vi "GSP_Logger_Handler.vi"(4 "error in (no error)":errorcluster, 5 "Log":T1, 6 "Actions":T2(ring), 7 "Log File Path":path) -> (0 "error out":errorcluster)   [LabVIEW 2015]
doc: "Provides an interface to the Logger thread. See the actions below.\n\nLaunch - launch the logger, supplying the path to the log file\n\nOpen - Show the logger's front panel\n\nClose - Hide the logger's front panel\n\nLog - Record the event supplied by Log control\n\nShutdown - Shutdown the logger thread"
uses:
  LogItem.ctl
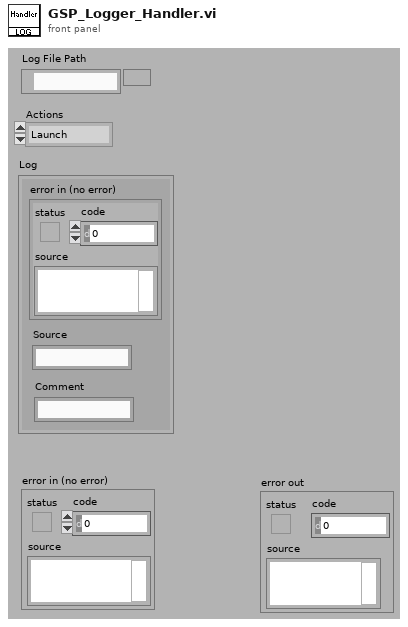
[diagram p1: front panel]
types:
  T1 = typedef "LogItem.ctl" = cluster{"error in (no error)":errorcluster, "Source":string, "Comment ":string}
  T2 = enum16{"Launch", "Log", "Open", "Close", "Shutdown"}
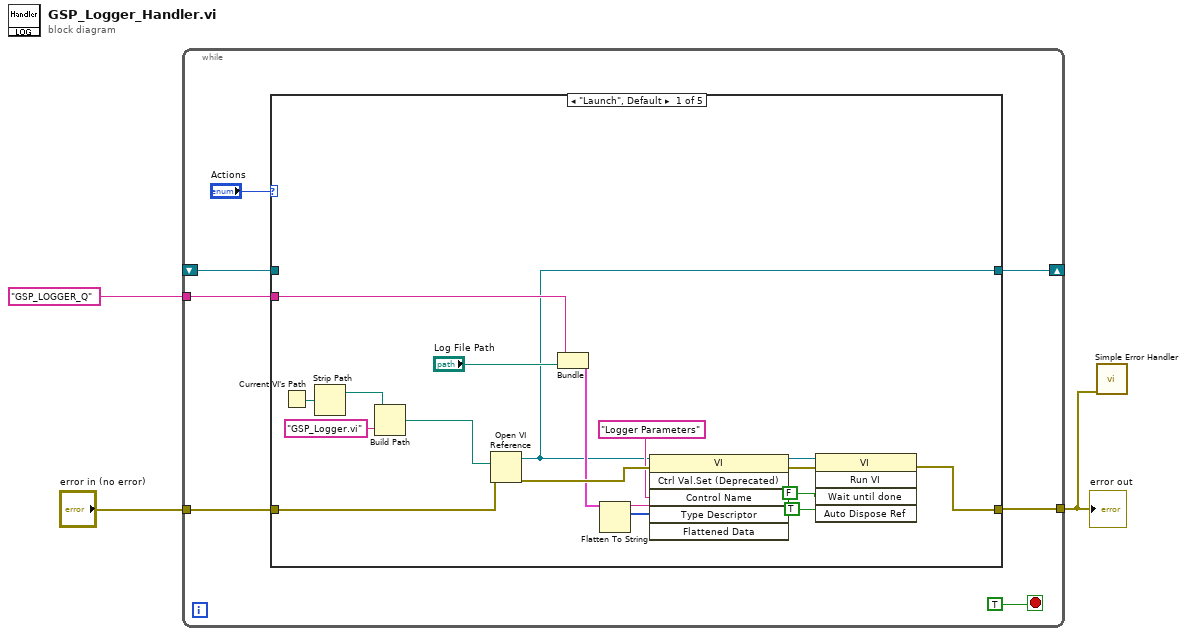
[diagram p0: block diagram]
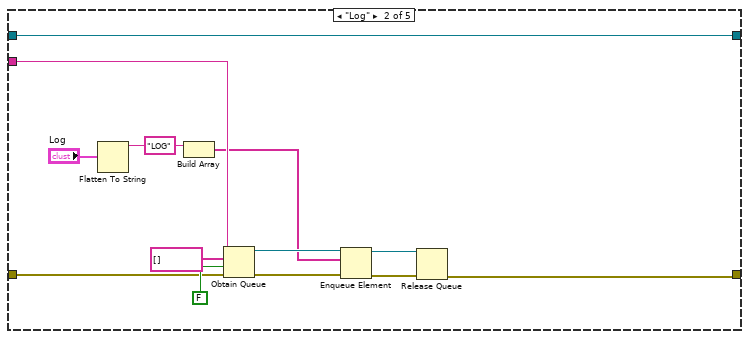
[diagram p2: hidden frame]
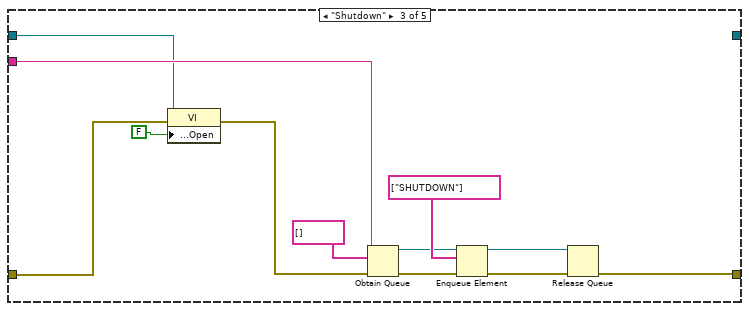
[diagram p3: hidden frame]
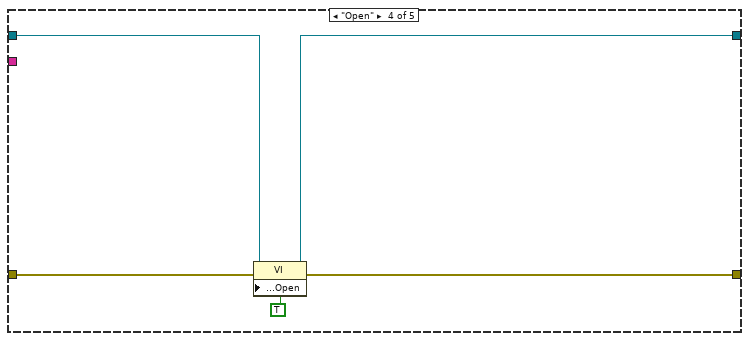
[diagram p4: hidden frame]
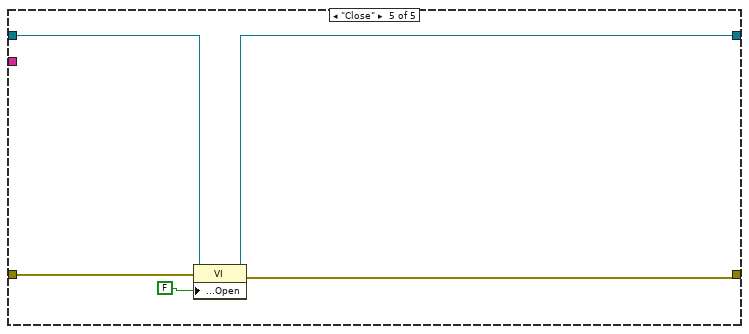
[diagram p5: hidden frame]
diagram:
  n1 = while {
    tunnel: "error in (no error)" -> [w7]
    tunnel: [w8] -> w1
    tunnel: "GSP_LOGGER_Q" -> [w6]
    shift-right: [w5] -> _
    shift-left: _ -> [w4]
    stop <- TRUE stop-if-true
    n2 = case shown="\"Launch\", Default" "Actions" {
      tunnel: w7 -> [w12 w40 w47 w58 w63]
      tunnel: [w14 w29 w43 w57 w60] -> w8
      tunnel: w6 -> [w13 w39 w52 _ _]
      tunnel: [w11 w32 _ w55 w61] -> w5
      tunnel: w4 -> [_ w32 w48 w56 w62]
      frame "Launch", Default {
        n3 = Current VI's Path() -> (path=w28:path)
        n4 = Strip Path(path=w28) -> (stripped path=w27:path)  [unwired: 1 out]
        n5 = Build Path(base path=w27, name or relative path="GSP_Logger.vi") -> (appended path=w25:path)
        n6 = Open VI Reference(vi path=w25, error in (no error)=w12) -> (vi reference=w11:refnum<vi>, error out=w24:errorcluster)  [unwired: 4 in]
        n7 = Bundle(w13, "Log File Path"="Log File Path") -> (w19:cluster{string, "Log File Path":path})  [unwired: 1 in]
        n8 = Flatten To String(anything=w19) -> (data string=w22:string, type string=w23:i16[])  [unwired: 3 in, 1 out]
        n9 = invoke class="VI" method="Ctrl Val.Set (Deprecated)"(reference=w11, error in=w24, "Control Name"="Logger Parameters", "Type Descriptor"=w23, "Flattened Data"=w22) -> (reference out=w18:refnum<vi>, error out=w17:errorcluster)  [unwired: 1 in, 4 out]
        n10 = invoke class="VI" method="Run VI"(reference=w18, error in=w17, "Wait until done"=FALSE, "Auto Dispose Ref"=TRUE) -> (error out=w14:errorcluster)  [unwired: 1 in, 4 out]
      }
      frame "Log" {
        n11 = Flatten To String(anything="Log") -> (data string=w35:string)  [unwired: 3 in, 2 out]
        n12 = Build Array("LOG" ("element"), w35) -> (w33:string[])
        n13 = Obtain Queue(name (unnamed)=w39, element data type=string[] [], create if not found? (T)=FALSE, error in (no error)=w40) -> (queue out=w38:refnum<queue>, error out=w37:errorcluster)  [unwired: 1 in, 1 out]
        n14 = Enqueue Element(queue=w38, element=w33, error in (no error)=w37) -> (queue out=w31:refnum<queue>, error out=w30:errorcluster)  [unwired: 1 in, 1 out]
        n15 = Release Queue(queue=w31, error in (no error)=w30) -> (error out=w29:errorcluster)  [unwired: 1 in, 2 out]
      }
      frame "Shutdown" {
        n16 = property class="VI"(reference=w48, error in=w47, "Front Panel Window:Open"=FALSE) -> (error out=w46:errorcluster)  [unwired: 1 out]
        n17 = Obtain Queue(name (unnamed)=w52, element data type=string[] [], error in (no error)=w46) -> (queue out=w50:refnum<queue>, error out=w51:errorcluster)  [unwired: 2 in, 1 out]
        n18 = Enqueue Element(queue=w50, element=string[] ["SHUTDOWN"], error in (no error)=w51) -> (queue out=w45:refnum<queue>, error out=w44:errorcluster)  [unwired: 1 in, 1 out]
        n19 = Release Queue(queue=w45, error in (no error)=w44) -> (error out=w43:errorcluster)  [unwired: 1 in, 2 out]
      }
      frame "Open" {
        n20 = property class="VI"(reference=w56, error in=w58, "Front Panel Window:Open"=TRUE) -> (reference out=w55:refnum<vi>, error out=w57:errorcluster)
      }
      frame "Close" {
        n21 = property class="VI"(reference=w62, error in=w63, "Front Panel Window:Open"=FALSE) -> (reference out=w61:refnum<vi>, error out=w60:errorcluster)
      }
    }
  }
  "error out" <- w1
  n22 = call <vilib>:"Simple Error Handler.vi"("error in (no error)"=w1) -> ()  [unwired: 4 in, 5 out]
